vi "VG_VCellMax70.vi"() -> ()   [LabVIEW 2020]
panel:
  out "VCellMax70":dbl
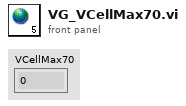
[diagram p1: front panel]
diagram:
